vi "Get Created Aliases.vi"(11 "Base Addresses Strategy in":refnum<class "Base Addresses Strategy.lvclass">) -> (2 "Created Aliases":string[](array[string]))   [LabVIEW 2021, in "jettl.lvlib" / "Addresses Strategy.lvlib" / "Base Addresses Strategy.lvclass"]
uses:
  Base Addresses Strategy.lvclass
  Base Addresses Strategy.lvclass/Base Addresses Strategy.ctl
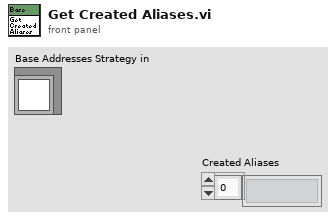
[diagram p1: front panel]
types:
  T1 = typedef "jettl.lvlib/Addresses Strategy.lvlib/Created.ctl" = map{string, refnum<class "Msg Type Strategy.lvclass">}
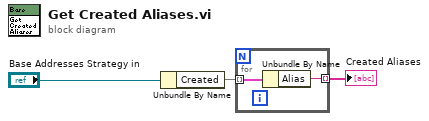
[diagram p0: block diagram]
diagram:
  n1 = Unbundle By Name("Base Addresses Strategy in") -> ("Created"=w1:T1)
  n2 = for {
    tunnel: [w4] -> w3 mode=indexing
    tunnel: w1 -> [w5] mode=indexing
    n3 = Unbundle By Name(w5) -> ("Alias"=w4:string)
  }
  "Created Aliases" <- w3
